vi "get_center.vi"(8 "error in (no error)":errorcluster, 11 "TrajectoryDL110420DoubleCircle in":refnum<class "TrajectoryDL110420DoubleCircle.lvclass">) -> (0 "error out":errorcluster, 2 "center":refnum<class "SpaceVector.lvclass">, 3 "TrajectoryDL110420DoubleCircle out":refnum<class "TrajectoryDL110420DoubleCircle.lvclass">)   [LabVIEW 2010, in "TrajectoryDL110420DoubleCircle.lvclass"]
uses:
  TrajectoryDL110420DoubleCircle.lvclass
  common/classes/SpaceVector/SpaceVector/SpaceVector.lvclass
  TrajectoryDL110420DoubleCircle.lvclass/TrajectoryDL110420DoubleCircle.ctl
  <vilib>/Analysis/baseanly.llb/Matrix Type of Inverse Matrix.ctl
  <vilib>/Analysis/7linalg.llb/Solve Linear Equations (single right hand).vi
  <vilib>/Analysis/7linalg.llb/Solve Linear Eqs (General).vi
  <vilib>/Analysis/7linalg.llb/Solve Linear Eqs (Gen, single right hand).vi
  <vilib>/Analysis/NI_AALPro.lvlib
  <vilib>/Analysis/NI_AALBase.lvlib
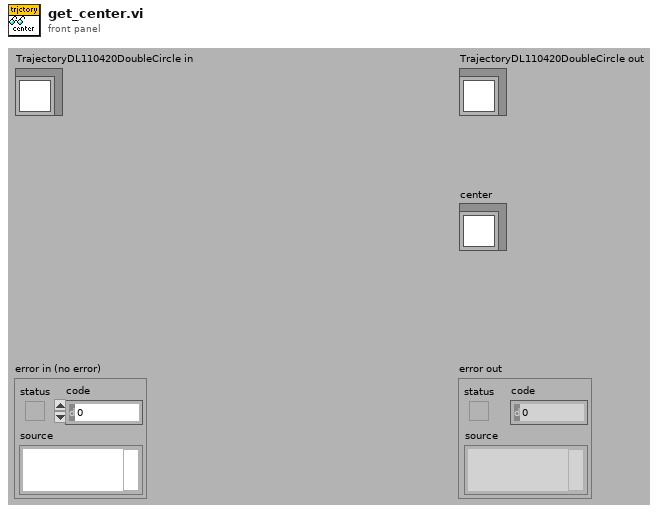
[diagram p1: front panel]
types:
  T1 = typedef "NI_AALBase.lvlib/Matrix Type of Inverse Matrix.ctl" = enum32{"General", "Positive Definite", "Lower Triangular", "Upper Triangular"}
  T2 = typedef "center_type_enum.ctl" = enum16{"midline", "centroid"}
  T3 = cluster{"[0]":refnum<class "SpaceVector.lvclass">, "[1]":refnum<class "SpaceVector.lvclass">, "[2]":refnum<class "SpaceVector.lvclass">}
  T4 = typedef "NI_Matrix.lvlib/RealMatrix.ctl" = dbl[][]
  T5 = cluster{"[0]":dbl[unit], "[1]":dbl[unit], "[2]":dbl[unit], "[3]":dbl[unit]}
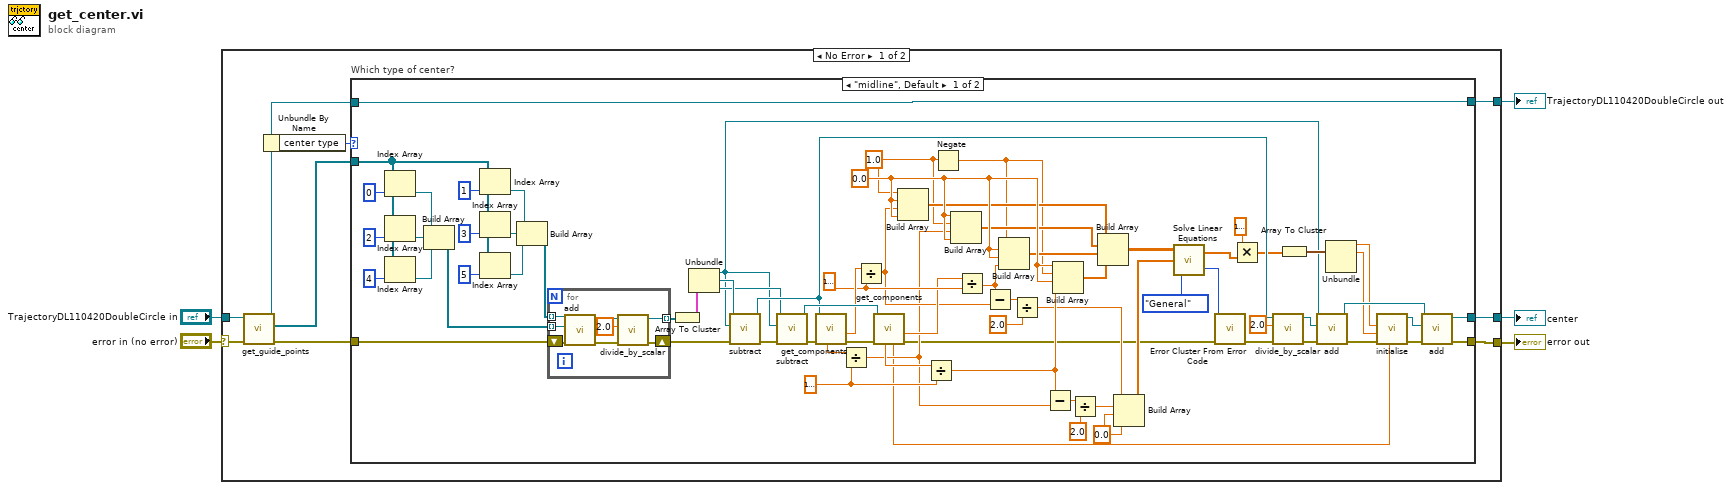
[diagram p0: block diagram]
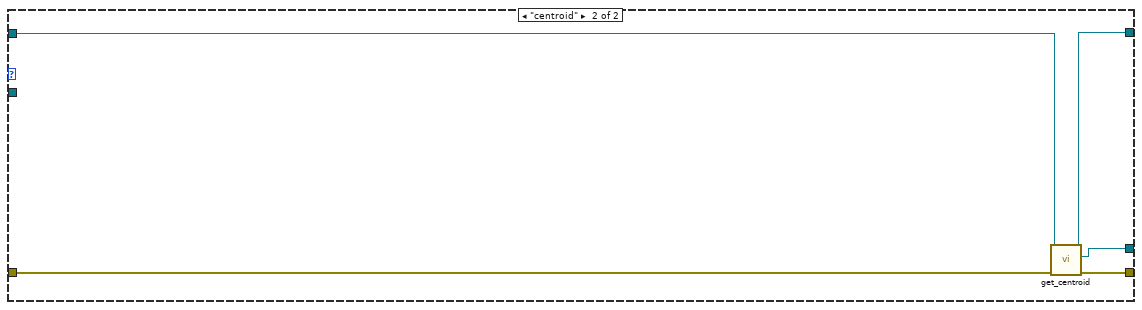
[diagram p2: hidden frame]
diagram:
  n1 = case shown="No Error" "error in (no error)" {
    selector: "error in (no error)" -> [w10 w103]
    tunnel: [w14 w103] -> w4
    tunnel: [w11 w102] -> w2
    tunnel: "TrajectoryDL110420DoubleCircle in" -> [w7 w102]
    tunnel: [w13 _] -> w1
    frame No Error {
      n2 = call-dynamic "get_guide_points.vi"("error in (no error)"=w10, "TrajectoryDL110420DoubleCircle in"=w7) -> ("error out"=w9:errorcluster, "guide points"=w6:refnum<class "SpaceVector.lvclass">[], "TrajectoryDL110420DoubleCircle out"=w8:refnum<class "TrajectoryDL110420DoubleCircle.lvclass">)  [unwired: 7 in]
      n3 = Unbundle By Name(w8) -> ("center type"=w12:T2)
      n4 = case "Which type of center?" shown="\"midline\", Default" w12 {
        tunnel: w6 -> [w76 _]
        tunnel: w9 -> [w73 w99]
        tunnel: [w31 w101] -> w14
        tunnel: [w30 w100] -> w13
        tunnel: w8 -> [w19 w98]
        tunnel: [w19 w97] -> w11
        frame "midline", Default {
          w43 = 0.0 ("element")
          w57 = dbl[unit] 1e-06 ("element")
          w56 = dbl[unit] 1e-06 ("element")
          w65 = 0.0 ("element")
          w39 = 1.0 ("element")
          n5 = Index Array(array=w76, index=0) -> (element=w82:refnum<class "SpaceVector.lvclass">)
          n6 = Index Array(array=w76, index=2) -> (element=w81:refnum<class "SpaceVector.lvclass">)
          n7 = Index Array(array=w76, index=4) -> (element=w80:refnum<class "SpaceVector.lvclass">)
          n8 = Build Array(w82, w81, w80) -> (w74:refnum<class "SpaceVector.lvclass">[])
          n9 = Index Array(array=w76, index=1) -> (element=w79:refnum<class "SpaceVector.lvclass">)
          n10 = Index Array(array=w76, index=3) -> (element=w78:refnum<class "SpaceVector.lvclass">)
          n11 = Index Array(array=w76, index=5) -> (element=w77:refnum<class "SpaceVector.lvclass">)
          n12 = Build Array(w79, w78, w77) -> (w75:refnum<class "SpaceVector.lvclass">[])
          n13 = for {
            tunnel: w75 -> [w95] mode=indexing
            tunnel: w74 -> [w94] mode=indexing
            tunnel: [w90] -> w72 mode=indexing
            shift-right: [w89] -> w69
            shift-left: w73 -> [w96]
            n14 = call "add.vi"("error in (no error)"=w96, "vector to be added"=w94, "SpaceVector in"=w95) -> ("error out"=w93:errorcluster, "SpaceVector out"=w92:refnum<class "SpaceVector.lvclass">)  [unwired: 7 in]
            n15 = call "divide_by_scalar.vi"("error in (no error)"=w93, "divisor"=2.0, "SpaceVector in"=w92) -> ("error out"=w89:errorcluster, "SpaceVector out"=w90:refnum<class "SpaceVector.lvclass">)  [unwired: 7 in]
          }
          n16 = Array To Cluster(array=w72) -> (cluster=w71:T3)
          n17 = Unbundle(w71) -> ("[0]"=w15:refnum<class "SpaceVector.lvclass">, "[1]"=w17:refnum<class "SpaceVector.lvclass">, "[2]"=w16:refnum<class "SpaceVector.lvclass">)
          n18 = call "subtract.vi"("error in (no error)"=w69, "subtrahend"=w15, "SpaceVector in"=w17) -> ("error out"=w70:errorcluster, "SpaceVector out"=w37:refnum<class "SpaceVector.lvclass">)  [unwired: 7 in]
          n19 = call "subtract.vi"("error in (no error)"=w70, "subtrahend"=w15, "SpaceVector in"=w16) -> ("error out"=w67:errorcluster, "SpaceVector out"=w66:refnum<class "SpaceVector.lvclass">)  [unwired: 7 in]
          n20 = call "get_components.vi"("error in (no error)"=w67, "SpaceVector in"=w37) -> ("error out"=w68:errorcluster, "x"=w60:dbl[unit], "y"=w59:dbl[unit])  [unwired: 4 in, 3 out]
          n21 = Divide(x=w59, y=w57) -> (x/y=w48:dbl)
          n22 = Divide(x=w60, y=w56) -> (x/y=w53:dbl)
          n23 = call "get_components.vi"("error in (no error)"=w68, "SpaceVector in"=w66) -> ("error out"=w40:errorcluster, "x"=w54:dbl[unit], "z"=w20:dbl[unit], "y"=w58:dbl[unit])  [unwired: 4 in, 2 out]
          n24 = Build Array(w39, w65, w53, w65) -> (w64:dbl[])
          n25 = Divide(x=w58, y=w57) -> (x/y=w49:dbl)
          n26 = Negate(x=w39) -> (-x=w38:dbl)
          n27 = Build Array(w65, w39, w48, w65) -> (w63:dbl[])
          n28 = Divide(x=w54, y=w56) -> (x/y=w52:dbl)
          n29 = Subtract(x=w52, y=w53) -> (x-y=w51:dbl)
          n30 = Build Array(w38, w65, w65, w52) -> (w62:dbl[])
          n31 = Divide(x=w51, y=2.0) -> (x/y=w45:dbl)
          n32 = Subtract(x=w49, y=w48) -> (x-y=w46:dbl)
          n33 = Build Array(w65, w38, w65, w49) -> (w61:dbl[])
          n34 = Divide(x=w46, y=2.0) -> (x/y=w44:dbl)
          n35 = Build Array(w64, w63, w62, w61) -> (w18:T4)
          n36 = Build Array(w45, w44, w43, w43) -> (w42:dbl[])
          n37 = call-poly <vilib>:"Solve Linear Equations.vi"("matrix type"=Matrix_Type_of_Inverse_Matrix."General", "Known Vector"=w42, "Input Matrix"=w18) -> ("error"=w41:i32, "Solution Vector"=w25:dbl[])
          n38 = call <vilib>:"Error Cluster From Error Code.vi"("error in (no error)"=w40, "error code (0)"=w41) -> ("error out"=w35:errorcluster)  [unwired: 7 in]
          n39 = Multiply(x=dbl[unit] 1e-06 ("element"), y=w25) -> (x*y=w24:dbl[unit][])
          n40 = call "divide_by_scalar.vi"("error in (no error)"=w35, "divisor"=2.0, "SpaceVector in"=w37) -> ("error out"=w33:errorcluster, "SpaceVector out"=w34:refnum<class "SpaceVector.lvclass">)  [unwired: 7 in]
          n41 = Array To Cluster(array=w24) -> (cluster=w26:T5)
          n42 = call "add.vi"("error in (no error)"=w33, "vector to be added"=w34, "SpaceVector in"=w15) -> ("error out"=w29:errorcluster, "SpaceVector out"=w32:refnum<class "SpaceVector.lvclass">)  [unwired: 7 in]
          n43 = Unbundle(w26) -> ("[0]"=w22:dbl[unit], "[1]"=w21:dbl[unit])  [unwired: 2 out]
          n44 = call "initialise.vi"("z"=w20, "error in (no error)"=w29, "y"=w21, "x"=w22) -> ("error out"=w28:errorcluster, "SpaceVector out"=w27:refnum<class "SpaceVector.lvclass">)  [unwired: 6 in]
          n45 = call "add.vi"("error in (no error)"=w28, "vector to be added"=w27, "SpaceVector in"=w32) -> ("error out"=w31:errorcluster, "SpaceVector out"=w30:refnum<class "SpaceVector.lvclass">)  [unwired: 7 in]
        }
        frame "centroid" {
          n46 = call-dynamic "get_centroid.vi"("error in (no error)"=w99, "TrajectoryDL110420DoubleCircle in"=w98) -> ("error out"=w101:errorcluster, "centroid"=w100:refnum<class "SpaceVector.lvclass">, "TrajectoryDL110420DoubleCircle out"=w97:refnum<class "TrajectoryDL110420DoubleCircle.lvclass">)  [unwired: 7 in]
        }
      }
    }
    frame Error {
    }
  }
  "error out" <- w4
  "TrajectoryDL110420DoubleCircle out" <- w2
  "center" <- w1
